vi "prepareStiffnessBaseline.vi"(8 "error in (no error)":errorcluster, 11 "Model in":refnum<class "Model.lvclass">) -> (0 "error out":errorcluster, 3 "Model out":refnum<class "Model.lvclass">)   [LabVIEW 2013, in "Model.lvclass"]
uses:
  Model.lvclass
  Model.lvclass/Model.ctl
  ApplicationElements/DistanceGauge/DistanceGauge.lvclass/DistanceGauge.ctl
  ApplicationElements/ForceSensor/ForceSensor.lvclass/ForceSensor.ctl
  ApplicationElements/Encoder/Encoder.lvclass/Encoder.ctl
  ApplicationElements/StiffnessMonitor/StiffnessMonitor.lvclass
  ApplicationElements/ForceSensor/ForceSensor.lvclass
  ApplicationElements/Encoder/Encoder.lvclass
  ApplicationElements/DistanceGauge/DistanceGauge.lvclass
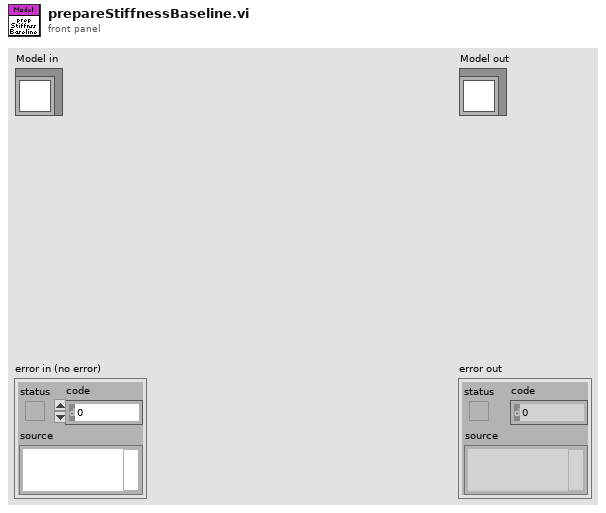
[diagram p1: front panel]
types:
  T1 = typedef "M2AADTTypedefs.lvlib/Distance Data.ctl" = cluster{"Distance Measured 1":dbl[unit], "Distance Measured 2":dbl[unit]}
  T2 = typedef "M2AADTTypedefs.lvlib/ForceDemand.ctl" = dbl[unit]
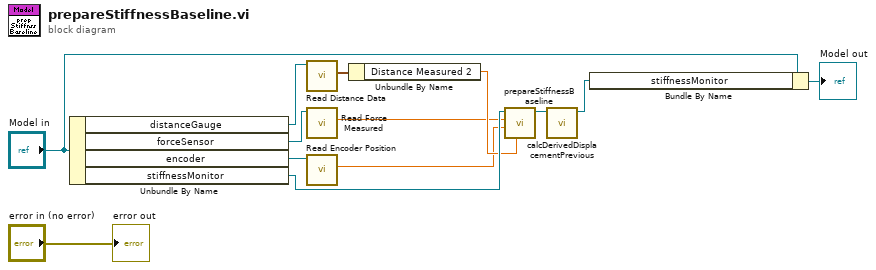
[diagram p0: block diagram]
diagram:
  n1 = Unbundle By Name("Model in") -> ("distanceGauge"=w2:refnum<class "DistanceGauge.lvclass">, "forceSensor"=w9:refnum<class "ForceSensor.lvclass">, "encoder"=w7:refnum<class "Encoder.lvclass">, "stiffnessMonitor"=w12:refnum<class "StiffnessMonitor.lvclass">)
  n2 = call "Read Distance Data.vi"("DistanceGauge in"=w2) -> ("Distance Data"=w1:T1)  [unwired: 9 in, 1 out]
  n3 = call "Read Force Measured.vi"("ForceSensor in"=w9) -> ("Force Demand"=w8:T2)  [unwired: 9 in, 1 out]
  n4 = call "Read Encoder Position.vi"("Encoder in"=w7) -> ("Encoder Position"=w6:dbl[unit])  [unwired: 9 in, 1 out]
  n5 = Unbundle By Name(w1) -> ("Distance Measured 2"=w10:dbl[unit])
  n6 = call "prepareStiffnessBaseline.vi"("Distance to Plate Measured"=w10, "Encoder Position"=w6, "Force Measured"=w8, "StiffnessMonitor in"=w12) -> ("StiffnessMonitor out"=w11:refnum<class "StiffnessMonitor.lvclass">)  [unwired: 6 in, 1 out]
  n7 = call "calcDerivedDisplacementPrevious.vi"("StiffnessMonitor in"=w11) -> ("StiffnessMonitor out"=w5:refnum<class "StiffnessMonitor.lvclass">)  [unwired: 9 in, 1 out]
  n8 = Bundle By Name(cluster="Model in", "stiffnessMonitor"=w5) -> (→"Model out":refnum<class "Model.lvclass">)
  "error out" <- "error in (no error)"
